vi "Laurel Handle Modbus Error.vi"(8 "error in (no error)":errorcluster, 10 "Remote IP Address":string="10.2.0.14", 11 "Modbus Master in":refnum<class "Modbus Master.lvclass">) -> (0 "error out":errorcluster, 3 "Modbus Master out":refnum<class "Modbus Master.lvclass">)   [LabVIEW 2020]
uses:
  <vilib>/NI/Modbus Library/API/Master/Modbus Master.lvclass
  <vilib>/NI/Modbus Library/API/Wrapper/Create TCP Master.vi
  <vilib>/NI/Modbus Library/API/Wrapper/API Main.lvlib
panel:
  in  "connect timeout ms":i32=10000
  out "status":bool
  out "Count":dbl
  in  "Error?":bool
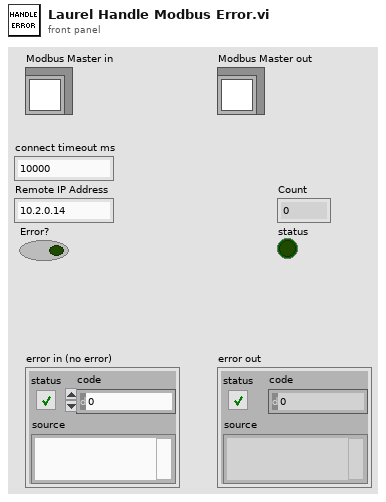
[diagram p1: front panel]
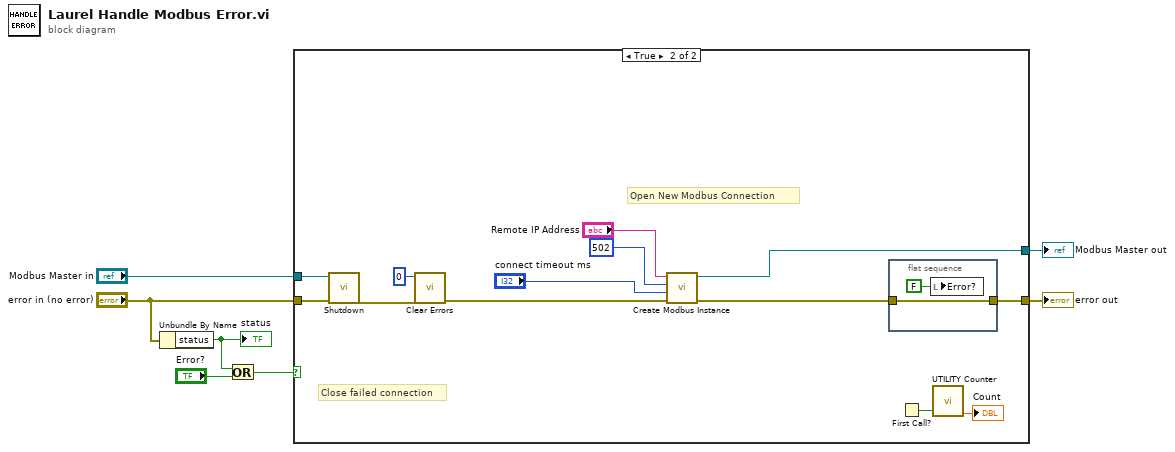
[diagram p0: block diagram]
diagram:
  n1 = Unbundle By Name("error in (no error)") -> ("status"=w4:bool)
  "status" <- w4
  n2 = Or(x=w4, y="Error?") -> (x .or. y?=w6:bool)
  n3 = case shown="True" w6 {
    tunnel: [w9 w22] -> w2
    tunnel: [w8 w18] -> w7
    tunnel: "Modbus Master in" -> [w9 w20]
    tunnel: "error in (no error)" -> [w8 w16]
    frame False {
    }
    frame True {
      # "Open New Modbus Connection"
      # "Close failed connection"
      n4 = call-dynamic "Shutdown.vi"("error in"=w16, "Modbus master in"=w20) -> ("error out"=w15:errorcluster)  [unwired: 9 in]
      n5 = call <vilib>:"Clear Errors.vi"("error in (no error)"=w15, "specific error code to clear (0: all)"=0) -> ("error out"=w13:errorcluster)  [unwired: 4 in, 1 out]
      n6 = call-poly <vilib>:"Create Modbus Instance.vi"("error in"=w13, "connect timeout ms"="connect timeout ms", "port (502)"=u16 502, "address"="Remote IP Address") -> ("error out"=w19:errorcluster, "TCP master instance"=w22:refnum<class "Modbus Master.lvclass">)  [unwired: 6 in]
      n7 = flat-sequence {
        tunnel: w19 -> [w24]
        tunnel: [w24] -> w18
        frame #0 {
          n8 = local write "Error?"(FALSE ("Error?")) -> ()
        }
      }
      n9 = First Call?() -> (First Call?: T/F=w21:bool)
      n10 = call "UTILITY Counter.vi"("Reset"=w21) -> ("Count"=→"Count":dbl)  [unwired: 10 in]
    }
  }
  "error out" <- w7
  "Modbus Master out" <- w2
